vi "Update Ongrid VF Device.vi"(7 "Global Configuration":T1={"Microgrid ID"=1, "VF Device ID"="", "Ongrid VF Priority"=[], "Offgrid VF Priority"=[], "AutoSwap Offgrid VF"=0, "AutoSwap Offgrid VF Delay (sec)"=0.0, "AutoSwap Resynch VF"=0, "PCC Device ID"="", "Device ID Array"=[], "Nominal Voltage"=0.0, "Nominal Frequency"=0.0, "Resynch Timeout (sec)"=0.0, "Island VF Activate Timeout (sec)"=90.0, "Island PCC Target Power (kW)"=0.0, "Island PCC Target Power Timeout (sec)"=0.0, "Island Grid Settle Time (sec)"=0.0, "Island PCC Failure Timeout (sec)"=0.0, "Activation Devices Present Timeout (sec)"=0.0, "Activation Devices Activated Timeout (sec)"=0.0, "Blackstart VF GenMode Wait (sec)"=0.0, "Blackstart VF DERCtrl Wait (sec)"=0.0, "Blackstart Success Wait (sec)"=0.0, "OnGrid Optimization Delay (sec)"=0.0, "OffGrid Optimization Delay (sec)"=0.0, "Resynch Frequency (Hz)"=0.0, "Optimization Path"=""}, 8 "error in":errorcluster, 11 "Resynchronization in":refnum<class "Resynchronization.lvclass">) -> (0 "error out":errorcluster, 3 "Resynchronization out":refnum<class "Resynchronization.lvclass">)   [LabVIEW 2018, in "Resynchronization Actor.lvlib" / "Resynchronization.lvclass"]
uses:
  Resynchronization.lvclass
  C:/Users/Administrator/Desktop/LabVIEW EMS/EMS Generic Actor/EMS Generic/EMS Generic.lvclass
  C:/Users/Administrator/Desktop/LabVIEW EMS/Device Communication and Control Abstract Actor/Device Communication and Control Abstract/Device Communication and Control Abstract.lvclass
  EMS Generic Actor/EMS Generic/Controls/Global Configuration.ctl
  <vilib>/ORNL/CSEISMIC DDS/CSEISMIC DDS Base/Data Types/Controls/DeviceID.ctl
  EMS Generic Actor/EMS Generic/EMS Generic.lvclass/EMS Generic.ctl
  <vilib>/ORNL/CSEISMIC DDS/CSEISMIC DDS Base/Data Types/DER_VF.ctl
  <vilib>/ActorFramework/Actor/Actor.lvclass/Actor.ctl
  Device Communication and Control Abstract Actor/Device Communication and Control Abstract/Device Communication and Control Abstract.lvclass/Device Communication and Control Abstract.ctl
  Device Communication and Control Abstract Actor/Device Communication and Control Abstract Messages/Set DER VF Msg/Set DER VF Msg.lvclass/Set DER VF Msg.ctl
  <vilib>/ActorFramework/Message Enqueuer/Message Enqueuer.lvclass/Message Enqueuer.ctl
  EMS Generic Actor/EMS Generic/Accessors - Global Configuration/Read Global Configuration.vi
  Device Communication and Control Abstract Actor/Device Communication and Control Abstract Messages/Set DER VF Msg/Send Set DER VF.vi
  <vilib>/ActorFramework/Actor/Read Caller Enqueuer.vi
  <vilib>/ActorFramework/Message Enqueuer/Enqueue.vi
  Device Communication and Control Abstract Actor/Device Communication and Control Abstract/Device Communication and Control Abstract.lvclass
  C:/Program Files (x86)/National Instruments/LabVIEW 2018/vi.lib/ActorFramework/Actor/Actor.lvclass
  Device Communication and Control Abstract Actor/Device Communication and Control Abstract Messages/Set DER VF Msg/Set DER VF Msg.lvclass
  C:/Program Files (x86)/National Instruments/LabVIEW 2018/vi.lib/ActorFramework/Message/Message.lvclass
  EMS Generic Actor/EMS Generic/Accessors - Global Configuration/Update Global Configuration.vi
  <vilib>/ActorFramework/Message Priority Queue/Priority Enqueue.vi
  EMS Generic Actor/EMS Generic/EMS Generic.lvclass
  <vilib>/ORNL/CSEISMIC DDS/CSEISMIC DDS Base/CSEISMIC DDS.lvclass
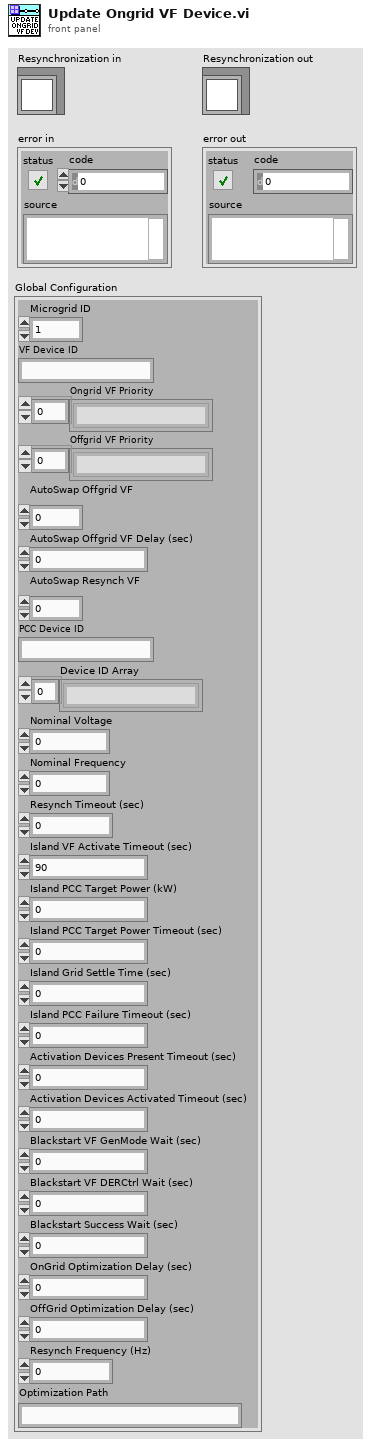
[diagram p1: front panel]
types:
  T1 = typedef "EMS Generic Actor.lvlib/EMS Generic.lvclass/Global Configuration.ctl" = cluster{"Microgrid ID":u8, "VF Device ID":T2, "Ongrid VF Priority":T2[], "Offgrid VF Priority":T2[], "AutoSwap Offgrid VF":u32, "AutoSwap Offgrid VF Delay (sec)":dbl, "AutoSwap Resynch VF":u32, "PCC Device ID":T2, "Device ID Array":T2[], "Nominal Voltage":dbl, "Nominal Frequency":dbl, "Resynch Timeout (sec)":dbl, "Island VF Activate Timeout (sec)":dbl, "Island PCC Target Power (kW)":dbl, "Island PCC Target Power Timeout (sec)":dbl, "Island Grid Settle Time (sec)":dbl, "Island PCC Failure Timeout (sec)":dbl, "Activation Devices Present Timeout (sec)":dbl, "Activation Devices Activated Timeout (sec)":dbl, "Blackstart VF GenMode Wait (sec)":dbl, "Blackstart VF DERCtrl Wait (sec)":dbl, "Blackstart Success Wait (sec)":dbl, "OnGrid Optimization Delay (sec)":dbl, "OffGrid Optimization Delay (sec)":dbl, "Resynch Frequency (Hz)":dbl, "Optimization Path":string}
  T2 = typedef "CSEISMIC DDS.lvlib/CSEISMIC DDS.lvclass/DeviceID.ctl" = string
  T3 = typedef "CSEISMIC DDS.lvlib/CSEISMIC DDS.lvclass/DER_VF.ctl" = cluster{"DeviceID":T2}
  T4 = typedef "EMS Generic Actor.lvlib/EMS Generic.lvclass/Data Type DVRs.ctl" = cluster{"IED_Status":refnum<data-value>, "IED_Status_0":refnum<data-value>, "DER_Measurement":refnum<data-value>, "DER_Info":refnum<data-value>, "DER_Status":refnum<data-value>, "ES_Measurement":refnum<data-value>, "ES_Info":refnum<data-value>, "PV_Info":refnum<data-value>, "SmartRelay_Info":refnum<data-value>, "SmartRelay_Measurement":refnum<data-value>, "Meter_Info":refnum<data-value>, "Meter_Measurement":refnum<data-value>, "HVAC_Status":refnum<data-value>, "HVAC_Measurement":refnum<data-value>, "PriceData_RealTime":refnum<data-value>, "PriceData_Demand":refnum<data-value>, "PriceData_Energy":refnum<data-value>, "ForecastData_Long":refnum<data-value>, "ForecastData_Short":refnum<data-value>, "DER_Control":refnum<data-value>, "DER_SetPointF":refnum<data-value>, "DER_SetPointP":refnum<data-value>, "DER_SetPointQ":refnum<data-value>, "DER_SetPointPF":refnum<data-value>, "DER_SetPointV":refnum<data-value>, "PV_setCurtailment":refnum<data-value>, "PV_setRampRate":refnum<data-value>, "Relay_Control":refnum<data-value>, "Load_Control":refnum<data-value>, "HVAC_Control":refnum<data-value>, "Generator_Info":refnum<data-value>, "ForecastData_Long_Backup":refnum<data-value>, "PriceData_RealTime_Backup":refnum<data-value>}
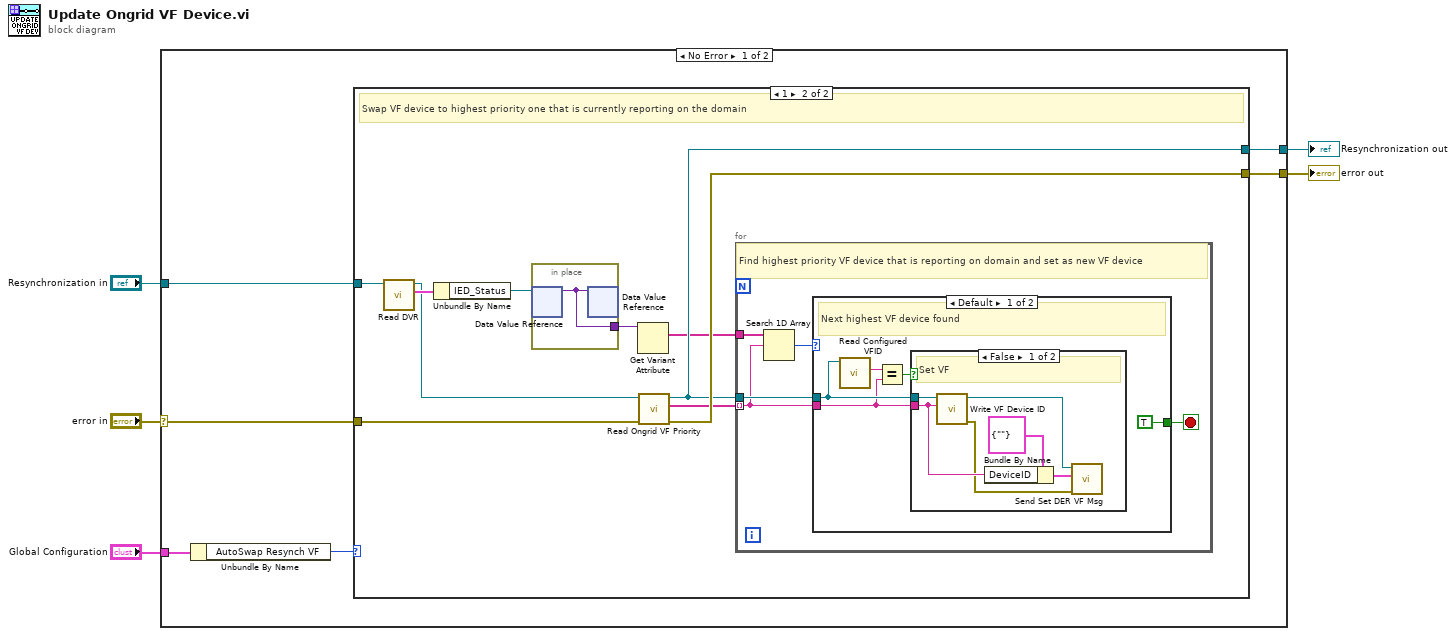
[diagram p0: block diagram]
diagram:
  n1 = case shown="No Error" "error in" {
    selector: "error in" -> [w8 w41]
    tunnel: [w11 w42] -> w5
    tunnel: "Resynchronization in" -> [w10 w42]
    tunnel: [w9 w41] -> w3
    tunnel: "Global Configuration" -> [w7 _]
    frame No Error {
      n2 = Unbundle By Name(w7) -> ("AutoSwap Resynch VF"=w6:u32)
      n3 = case shown="1" w6 {
        tunnel: [w13 w19] -> w11
        tunnel: w10 -> [w13 w15]
        tunnel: [w12 w23] -> w9
        tunnel: w8 -> [w12 w22]
        frame 0, Default {
          # "Either we're not auto swapping or it's not yet time to swap.  Do nothing."
        }
        frame 1 {
          # "Swap VF device to highest priority one that is currently reporting on the domain"
          n4 = call "Read DVR.vi"("EMS Generic in"=w15) -> ("DVR"=w21:T4, "EMS Generic out"=w14:refnum<class "Resynchronization.lvclass">)  [unwired: 9 in]
          n5 = Unbundle By Name(w21) -> ("IED_Status"=w18:refnum<data-value>)
          n6 = in-place {
            in-place-border: [w24] -> w17
            n7 = in-place-dvr #1(w18) -> (w24:variant)  [unwired: 1 out]
            n8 = in-place-dvr #1(w24) -> ()  [unwired: 2 out]
          }
          n9 = Get Variant Attribute(Variant=w17) -> (names=w16:string[])  [unwired: 3 in, 3 out]
          n10 = call "Read Ongrid VF Priority.vi"("error in"=w22, "EMS Generic in"=w14) -> ("error out"=w23:errorcluster, "Ongrid VF Priority"=w20:T2[], "EMS Generic out"=w19:refnum<class "Resynchronization.lvclass">)  [unwired: 7 in]
          n11 = for {
            tunnel: w20 -> [w26] mode=indexing
            tunnel: w16 -> [w29]
            tunnel: w19 -> [w27]
            stop <- w25 stop-if-true
            # "Find highest priority VF device that is reporting on domain and set as new VF device"
            n12 = Search 1D Array(1D array=w29, element=w26) -> (index of element=w28:i32)  [unwired: 1 in]
            n13 = case shown="Default" w28 {
              tunnel: w27 -> [w33 _]
              tunnel: w26 -> [w31 _]
              tunnel: [TRUE _] -> w25
              frame Default {
                # "Next highest VF device found"
                n14 = call "Read Configured VFID.vi"("EMS Generic in"=w33) -> ("VFID"=w32:T2)  [unwired: 8 in, 2 out]
                n15 = Equal?(x=w32, y=w31) -> (x = y?=w30:bool)
                n16 = case shown="False" w30 {
                  tunnel: w31 -> [w37 _]
                  tunnel: w33 -> [w40 _]
                  frame False {
                    # "Set VF"
                    n17 = call "Write VF Device ID.vi"("VF Device"=w37, "EMS Generic in"=w40) -> ("error out"=w35:errorcluster, "EMS Generic out"=w36:refnum<class "Resynchronization.lvclass">)  [unwired: 8 in]
                    n18 = Bundle By Name(cluster=T3 {"DeviceID"=""} ("DER_VF"), "DeviceID"=w37) -> (w38:T3)
                    n19 = call "Send Set DER VF Msg.vi"("error in"=w35, "DER_VF"=w38, "SCADA Sub Abstract in"=w36) -> ()  [unwired: 7 in, 2 out]
                  }
                  frame True {
                    # "Already VF"
                  }
                }
              }
              frame -1 {
                # "Backup VF device not reporting on domain"
              }
            }
          }
        }
      }
    }
    frame Error {
    }
  }
  "Resynchronization out" <- w5
  "error out" <- w3
